vi "(SubVI)_Wrap_PID_AoWrite_Multivessels_for_test.vi"(2 "Input cluster":T1) -> (0 "output cluster":T2)   [LabVIEW 2019]
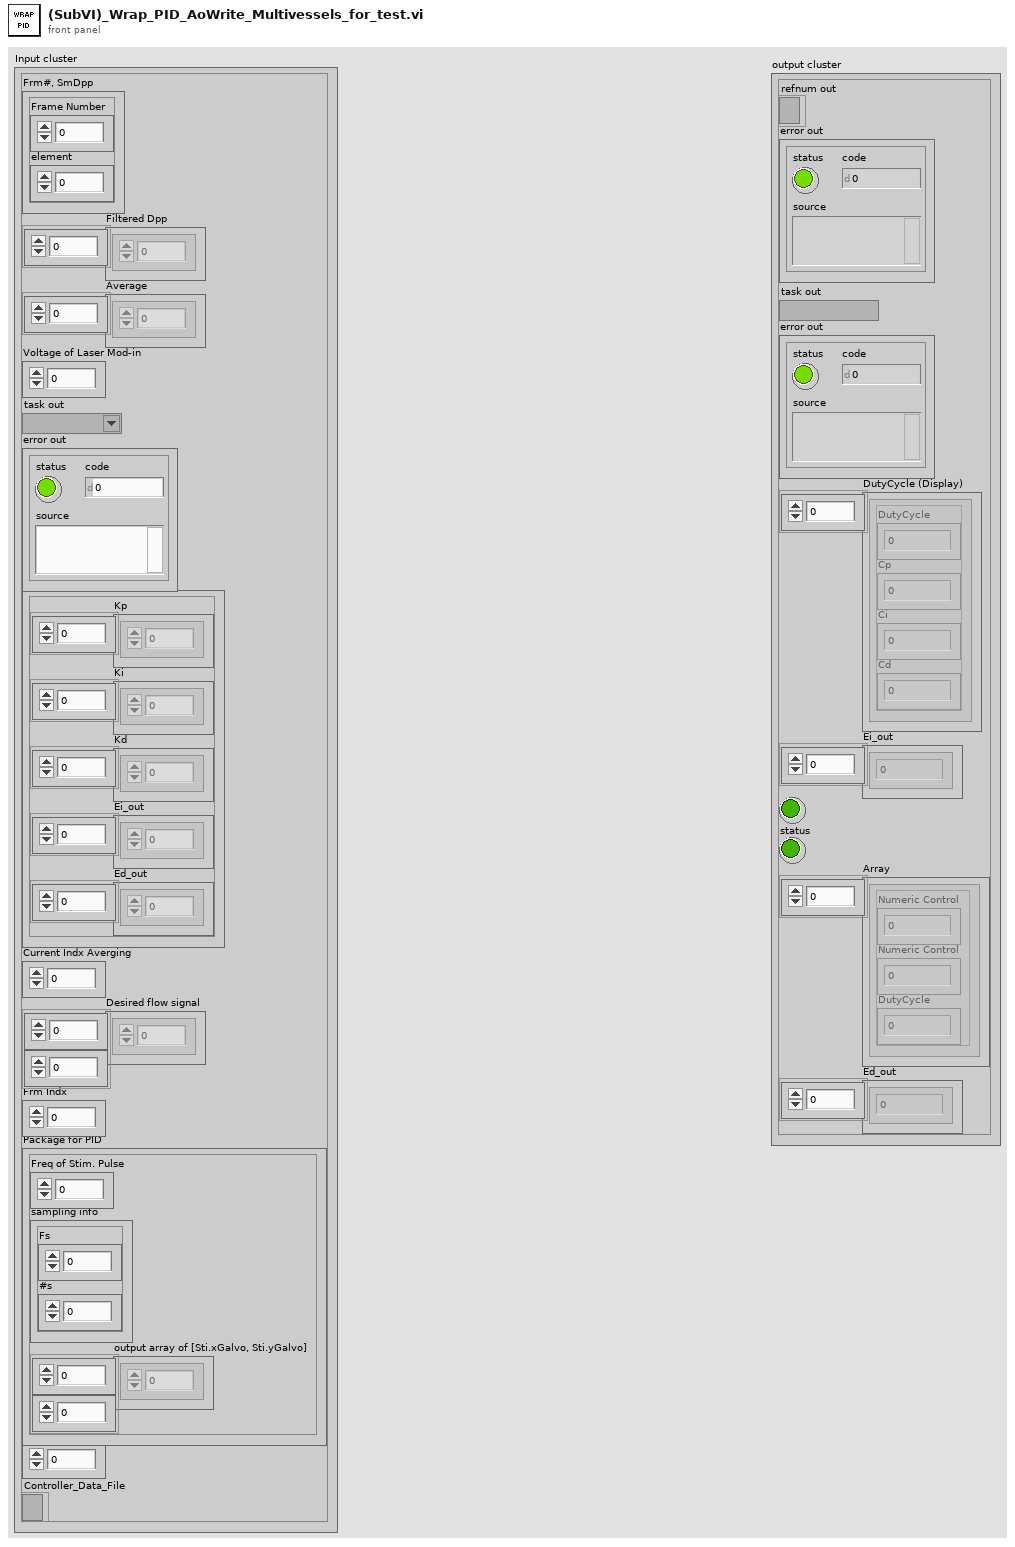
[diagram p1: front panel]
types:
  T1 = cluster{"Frm#, SmDpp":cluster{"Frame Number":dbl, "element":dbl}, "Filtered Dpp":dbl[], "Average":dbl[], "Voltage of Laser Mod-in":dbl, "task out":refnum<k21>, "error out":errorcluster, "Cluster":cluster{"Kp":dbl[], "Ki":dbl[], "Kd":dbl[], "Ei_out":dbl[], "Ed_out":dbl[]}, "Current Indx Averging":dbl, "Desired flow signal":dbl[][], "Frm Indx":dbl, "Package for PID":cluster{"Freq of Stim. Pulse":dbl, "sampling info":cluster{"Fs":dbl, "#s":dbl}, "output array of [Sti.xGalvo, Sti.yGalvo]":dbl[][]}, "Numeric Control":i32, "Controller_Data_File":refnum<file>}
  T2 = cluster{"refnum out":refnum<file>, "error out":errorcluster, "task out":refnum<k21>, "error out":errorcluster, "DutyCycle (Display)":cluster{"DutyCycle":dbl, "Cp":dbl, "Ci":dbl, "Cd":dbl}[], "Ei_out":dbl[], "Boolean":bool, "status":bool, "Array":cluster{"Numeric Control":dbl, "Numeric Control":dbl, "DutyCycle":dbl}[], "Ed_out":dbl[]}
  T3 = cluster{"Kp":dbl[], "Ki":dbl[], "Kd":dbl[], "Ei_out":dbl[], "Ed_out":dbl[]}
  T4 = cluster{"Freq of Stim. Pulse":dbl, "sampling info":cluster{"Fs":dbl, "#s":dbl}, "output array of [Sti.xGalvo, Sti.yGalvo]":dbl[][]}
  T5 = cluster{"Numeric Control":dbl, "Numeric Control":dbl, "DutyCycle":dbl}[]
  T6 = cluster{"DutyCycle":dbl, "Cp":dbl, "Ci":dbl, "Cd":dbl}[]
  T7 = cluster{dbl[], "Current Indx Averging":dbl, "Frame Number":dbl, "Desired flow signal":dbl[], "output KpKiKdEi":cluster{"Kp":dbl[], "Ki":dbl[], "Kd":dbl[]}, "DutyCycleArray":dbl[]}
  T8 = cluster{"refnum out":refnum<file>, "error out":errorcluster, "task out":refnum<k21>, "error out":errorcluster, "DutyCycle (Display)":cluster{"DutyCycle":dbl, "Cp":dbl, "Ci":dbl, "Cd":dbl}[], "Ei_out":dbl[], bool, "status":bool, "Array":cluster{"Numeric Control":dbl, "Numeric Control":dbl, "DutyCycle":dbl}[], "Ed_out":dbl[]}
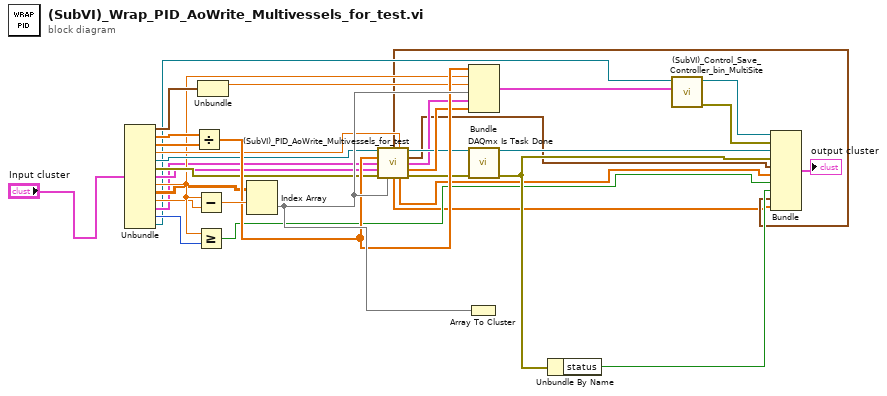
[diagram p0: block diagram]
diagram:
  n1 = Unbundle("Input cluster") -> ("Frm#, SmDpp"=w25:cluster{"Frame Number":dbl, "element":dbl}, "Filtered Dpp"=w24:dbl[], "Average"=w23:dbl[], "Voltage of Laser Mod-in"=w22:dbl, "task out"=w21:refnum<k21>, "error out"=w20:errorcluster, "Cluster"=w19:T3, "Current Indx Averging"=w18:dbl, "Desired flow signal"=w17:dbl[][], "Frm Indx"=w16:dbl, "Package for PID"=w15:T4, "Numeric Control"=w14:i32, "Controller_Data_File"=w13:refnum<file>)
  n2 = Divide(x=w24, y=w23) -> (x/y=w32:dbl[])
  n3 = Subtract(x=w18, y=w16) -> (x-y=w34:dbl)
  n4 = Greater Or Equal?(x=w18, y=w14) -> (x >= y?=w6:bool)
  n5 = Unbundle(w25) -> ("Frame Number"=w28:dbl)  [unwired: 1 out]
  n6 = Index Array(array=w17, index (row)=w34) -> (element=w33:dbl[])  [unwired: 1 in]
  n7 = call "(SubVI)_PID_AoWrite_Multivessels_for_test.vi"("task in"=w21, "amplitude"=w22, "Filtered Dpp"=w32, "Package from Galvo Pattern Generator"=w15, "KpKiKdEi"=w19, "error in"=w20, "Desired flow signal"=w33) -> ("Array"=w4:T5, "task out"=w30:refnum<k21>, "DutyCycle (Display)"=w8:T6, "output KpKiKdEi"=w26:cluster{"Kp":dbl[], "Ki":dbl[], "Kd":dbl[]}, "DutyCycleArray"=w31:dbl[], "Ed_out"=w3:dbl[], "Ei_out"=w7:dbl[], "error out"=w29:errorcluster)  [unwired: 1 in]
  n8 = Array To Cluster(array=w33) -> ()  [unwired: 1 out]
  n9 = Bundle(w32, "Current Indx Averging"=w18, "Frame Number"=w28, "Desired flow signal"=w33, "output KpKiKdEi"=w26, "DutyCycleArray"=w31) -> (w27:T7)  [unwired: 1 in]
  n10 = call <vilib>:"DAQmx Is Task Done.vi"("task/channels in"=w30, "error in"=w29) -> ("task out"=w10:refnum<k21>, "error out"=w9:errorcluster)  [unwired: 11 in, 1 out]
  n11 = Unbundle By Name(w9) -> ("status"=w5:bool)
  n12 = call "(SubVI)_Control_Save_Controller_bin_MultiSite.vi"("Input cluster"=w27, "refnum in"=w13) -> ("error out"=w11:errorcluster, "refnum out"=w12:refnum<file>)  [unwired: 8 in]
  n13 = Bundle("refnum out"=w12, "error out"=w11, "task out"=w10, "error out"=w9, "DutyCycle (Display)"=w8, "Ei_out"=w7, w6, "status"=w5, "Array"=w4, "Ed_out"=w3) -> (→"output cluster":T8)  [unwired: 1 in]
